vi "ExSubToggleFlip.vi"(2 "error in (no error)":errorcluster, 3 "Camera Handle":u32) -> (0 "error out":errorcluster, 1 "Camera Handle":u32)   [LabVIEW 2010]
uses:
  GlobalReverseFlag.vi
  GlobalFlipFlag.vi
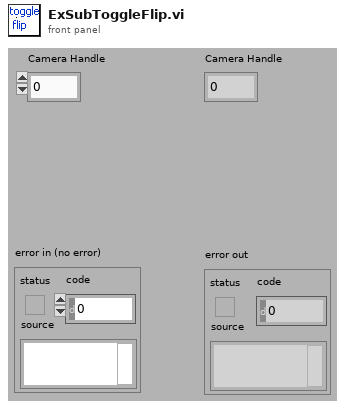
[diagram p1: front panel]
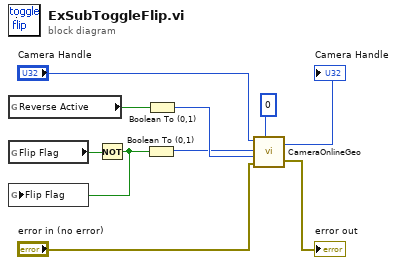
[diagram p0: block diagram]
diagram:
  n1 = global read "GlobalReverseFlag.vi" "Reverse Active"() -> (w3:bool)
  n2 = global read "GlobalFlipFlag.vi" "Flip Flag"() -> (w2:bool)
  n3 = Not(x=w2) -> (.not. x?=w1:bool)
  n4 = global write "GlobalFlipFlag.vi" "Flip Flag"(w1) -> ()
  n5 = Boolean To (0,1)(Boolean=w1) -> (0, 1=w5:i16)
  n6 = Boolean To (0,1)(Boolean=w3) -> (0, 1=w10:i16)
  n7 = call <userlib>:"CameraOnlineGeo.vi"("Camera Handle"="Camera Handle", "Flip Flag"=w5, "Reverse Flag"=w10, "error in"="error in (no error)", "Rotate Flag"=0) -> ("Camera Handle"=→"Camera Handle":u32, "error out"=→"error out":errorcluster)
